vi "PwF_ToF_CoreDeviceConfig.vi"(8 "NewDeviceID":u8, 11 "SNofDevToChange":u32) -> ()   [LabVIEW 2018]
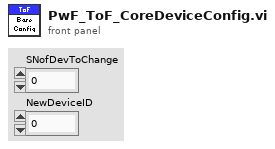
[diagram p1: front panel]
types:
  T1 = cluster{"upper limit":u8, u8, u8, u8, u8, u8, "NewDeviceID":u8}
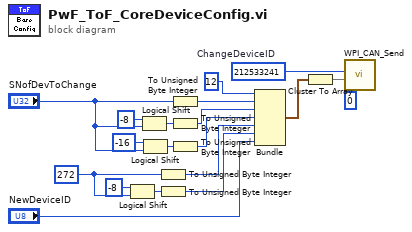
[diagram p0: block diagram]
diagram:
  w7 = u16 272 ("upper limit")
  w19 = u32 212533241  # ChangeDeviceID
  n1 = Logical Shift(y=i16 -8, x=w7) -> (x << y=w8:u16)
  n2 = Logical Shift(y=i16 -8, x="SNofDevToChange") -> (x << y=w14:u32)
  n3 = Logical Shift(y=i16 -16, x="SNofDevToChange") -> (x << y=w13:u32)
  n4 = To Unsigned Byte Integer(number=w7) -> (unsigned 8bit integer=w6:u8)
  n5 = To Unsigned Byte Integer(number=w8) -> (unsigned 8bit integer=w5:u8)
  n6 = To Unsigned Byte Integer(number="SNofDevToChange") -> (unsigned 8bit integer=w12:u8)
  n7 = To Unsigned Byte Integer(number=w14) -> (unsigned 8bit integer=w11:u8)
  n8 = To Unsigned Byte Integer(number=w13) -> (unsigned 8bit integer=w10:u8)
  n9 = Bundle("upper limit"=u8 12, w12, w11, w10, w6, w5, "NewDeviceID"="NewDeviceID") -> (w2:T1)  [unwired: 1 in]
  n10 = Cluster To Array(cluster=w2) -> (array=w3:u8[])
  n11 = call <vilib>:"WPI_CAN_Send.vi"("Period (ms)"=0, "Data"=w3, "Message ID"=w19) -> ()  [unwired: 8 in, 1 out]
